vi "connectSubData.vi"(8 "error in (no error)":errorcluster, 11 "MiddlewareSVThisComponent in":refnum<class "MiddlewareSVThisComponent.lvclass">) -> (0 "error out":errorcluster, 3 "MiddlewareSVThisComponent out":refnum<class "MiddlewareSVThisComponent.lvclass">)   [LabVIEW 2015, in "MiddlewareSVThisComponent.lvclass"]
uses:
  MiddlewareSVThisComponent.lvclass
  ComponentTemplateCore/ComponentModel/ComponentModel/Typedefs/CommunicationConfig.ctl
  ComponentTemplateCore/ComponentModel/ComponentModel/Typedefs/SVProcessConfig.ctl
  ComponentTemplateCore/ComponentModel/ComponentModelDT/ConfigurationFileReaderDT/ConfigurationFileReaderDT.lvclass
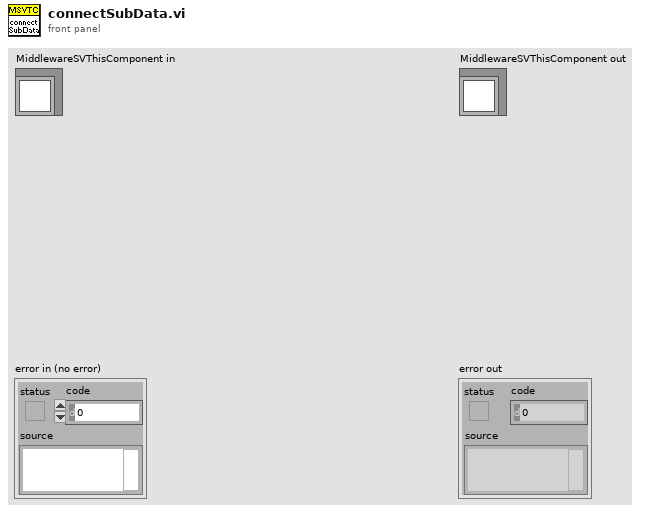
[diagram p1: front panel]
types:
  T1 = typedef "SVProcessConfig.ctl" = cluster{"subDataProcessPrototype":string, "pubDataProcessPrototype":string, "commandProcessPrototype":string, "commandSVName":string}
  T2 = typedef "CommunicationConfig.ctl" = cluster{"hostComputerAddress":string, "ComponentAcronym":string, "InstanceIdentifier":i32}
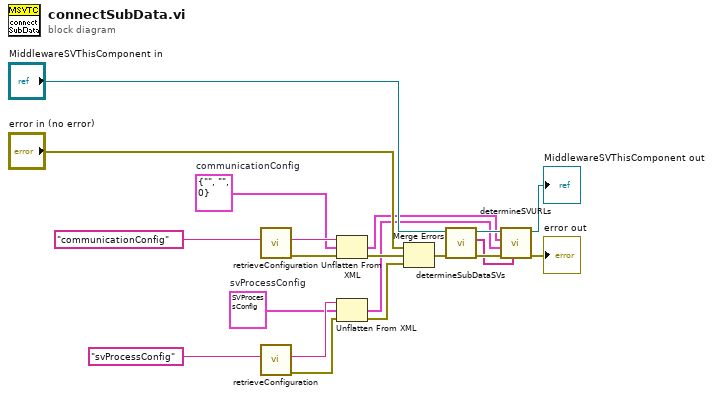
[diagram p0: block diagram]
diagram:
  w13 = T1 {"subDataProcessPrototype"="SubDataSV", "pubDataProcessPrototype"="PubDataSV", "commandProcessPrototype"="CommandSV", "commandSVName"="Command"}  # svProcessConfig
  w17 = T2 {"hostComputerAddress"="", "ComponentAcronym"="", "InstanceIdentifier"=0}  # communicationConfig
  n1 = call "retrieveConfiguration.vi"("dataName"="communicationConfig") -> ("error out"=w18:errorcluster, "dataValueFromFile"=w19:string)  [unwired: 8 in, 1 out]
  n2 = call "retrieveConfiguration.vi"("dataName"="svProcessConfig") -> ("error out"=w16:errorcluster, "dataValueFromFile"=w15:string)  [unwired: 8 in, 1 out]
  n3 = Unflatten From XML(xml string=w19, type=w17, error in (no error)=w18) -> (value=w5:T2, error out=w12:errorcluster)
  n4 = Unflatten From XML(xml string=w15, type=w13, error in (no error)=w16) -> (value=w4:T1, error out=w11:errorcluster)
  n5 = Merge Errors("error in (no error)", w12, w11) -> (w9:errorcluster)
  n6 = call "determineSubDataSVs.vi"("error in (no error)"=w9, "MiddlewareSVThisComponent in"="MiddlewareSVThisComponent in") -> ("error out"=w7:errorcluster, "svNames"=w1:string[], "MiddlewareSVThisComponent out"=w6:refnum<class "MiddlewareSVThisComponent.lvclass">)  [unwired: 7 in]
  n7 = call-dynamic "determineSVURLs.vi"("SVNames"=w1, "error in (no error)"=w7, "svProcessConfig"=w4, "communicationConfig"=w5, "MiddlewareSV in"=w6) -> ("error out"=→"error out":errorcluster, "MiddlewareSV out"=→"MiddlewareSVThisComponent out":refnum<class "MiddlewareSVThisComponent.lvclass">)  [unwired: 5 in]
